vi "Browse Options To Selection Mode.vi"(9 "Treat LLB's as Folders":bool, 10 "New or Existing":T2, 11 "Files or Folders":T3) -> (3 "Selection Mode":T1)   [LabVIEW 2018, in "Path Data Type.lvclass"]
uses:
  Path Data Type.lvclass
  Files or Folders.ctl
  New or Existing.ctl
  Selection Mode.ctl
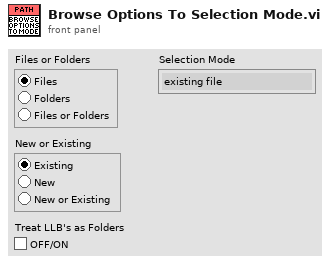
[diagram p1: front panel]
types:
  T1 = typedef "Path Data Type.lvclass/Selection Mode.ctl" = enum32{"existing file", "new file", "new or existing file", "existing dir", "new dir", "new or existing dir", "existing file (use LLBs)", "new file (use LLBs)", "new or existing file (use LLBs)", "new or existing file or directory (use LLBs)", "existing dir (use LLBs)", "new dir (use LLBs)", "new or existing dir (use LLBs)", "existing file or dir", "new file or dir", "new or existing file or dir", "existing file or dir (use LLBs)", "new file or dir (use LLBs)"}
  T2 = typedef "Path Data Type.lvclass/New or Existing.ctl" = enum32{"Existing", "New", "New or Existing"}
  T3 = typedef "Path Data Type.lvclass/Files or Folders.ctl" = enum32{"Files", "Folders", "Files or Folders"}
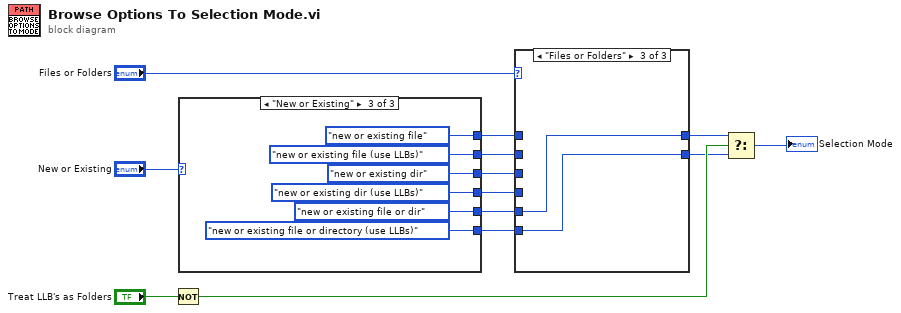
[diagram p0: block diagram]
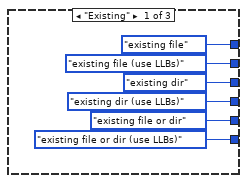
[diagram p4: hidden frame]
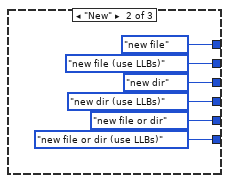
[diagram p5: hidden frame]
diagram:
  n1 = Not(x="Treat LLB's as Folders") -> (.not. x?=w3:bool)
  n2 = case shown="\"New or Existing\"" "New or Existing" {
    tunnel: [Selection_Mode."existing file" ("Selection Mode") Selection_Mode."new file" ("Selection Mode") Selection_Mode."new or existing file" ("Selection Mode")] -> w11
    tunnel: [Selection_Mode."existing file (use LLBs)" ("Selection Mode") Selection_Mode."new file (use LLBs)" ("Selection Mode") Selection_Mode."new or existing file (use LLBs)" ("Selection Mode")] -> w10
    tunnel: [Selection_Mode."existing dir" ("Selection Mode") Selection_Mode."new dir" ("Selection Mode") Selection_Mode."new or existing dir" ("Selection Mode")] -> w9
    tunnel: [Selection_Mode."existing dir (use LLBs)" ("Selection Mode") Selection_Mode."new dir (use LLBs)" ("Selection Mode") Selection_Mode."new or existing dir (use LLBs)" ("Selection Mode")] -> w8
    tunnel: [Selection_Mode."existing file or dir" ("Selection Mode") Selection_Mode."new file or dir" ("Selection Mode") Selection_Mode."new or existing file or dir" ("Selection Mode")] -> w7
    tunnel: [Selection_Mode."existing file or dir (use LLBs)" ("Selection Mode") Selection_Mode."new file or dir (use LLBs)" ("Selection Mode") Selection_Mode."new or existing file or directory (use LLBs)" ("Selection Mode")] -> w6
    frame "Existing" {
    }
    frame "New" {
    }
    frame "New or Existing" {
    }
  }
  n3 = case shown="\"Files or Folders\"" "Files or Folders" {
    tunnel: w11 -> [w33 _ _]
    tunnel: w10 -> [w32 _ _]
    tunnel: w9 -> [_ w35 _]
    tunnel: w8 -> [_ w34 _]
    tunnel: w7 -> [_ _ w37]
    tunnel: w6 -> [_ _ w36]
    tunnel: [w33 w35 w37] -> w2
    tunnel: [w32 w34 w36] -> w1
    frame "Files" {
    }
    frame "Folders" {
    }
    frame "Files or Folders" {
    }
  }
  n4 = Select(t=w2, s=w3, f=w1) -> (s? t:f=→"Selection Mode":T1)
